vi "FilterSixArray.vi"(11 "DesiredFM_FF":dbl[](array[numeric])) -> (3 "appended array":dbl[](array[numeric]))   [LabVIEW 2017]
uses:
  <vilib>/Analysis/3filter.llb/Filter Passband Type.ctl
  <vilib>/ptbypt/NI_PtbyPt.lvlib
  <vilib>/Analysis/NI_AALBase.lvlib
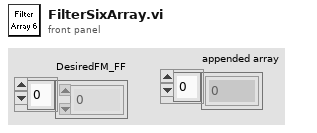
[diagram p1: front panel]
types:
  T1 = typedef "NI_AALBase.lvlib/Filter Passband Type.ctl" = enum32{"Lowpass", "Highpass", "Bandpass", "Bandstop"}
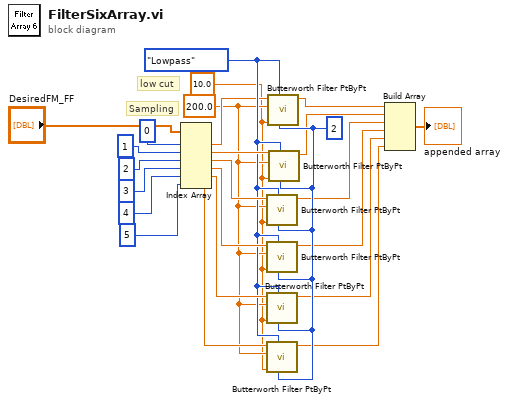
[diagram p0: block diagram]
diagram:
  w8 = 10.0 ("sampling freq: fs")
  w9 = 2 ("order")
  w10 = 200.0 ("sampling freq: fs")
  w12 = Filter_Passband_Type."Lowpass" ("filter type")
  # "Sampling"
  # "low cut"
  n1 = Index Array(array="DesiredFM_FF", index #1=0 ("index"), index #2=1 ("index"), index #3=2 ("index"), index #4=3 ("index"), index #5=4 ("index"), index #6=5 ("index")) -> (element #1=w11:dbl, element #2=w17:dbl, element #3=w16:dbl, element #4=w15:dbl, element #5=w14:dbl, element #6=w13:dbl)
  n2 = call <vilib>:"Butterworth Filter PtByPt.vi"("order"=w9, "filter type"=w12, "low cutoff freq: fl"=w8, "sampling freq: fs"=w10, "x"=w16) -> ("Filtered x"=w5:dbl)  [unwired: 4 in, 1 out]
  n3 = call <vilib>:"Butterworth Filter PtByPt.vi"("order"=w9, "filter type"=w12, "low cutoff freq: fl"=w8, "sampling freq: fs"=w10, "x"=w15) -> ("Filtered x"=w4:dbl)  [unwired: 4 in, 1 out]
  n4 = call <vilib>:"Butterworth Filter PtByPt.vi"("order"=w9, "filter type"=w12, "low cutoff freq: fl"=w8, "sampling freq: fs"=w10, "x"=w14) -> ("Filtered x"=w3:dbl)  [unwired: 4 in, 1 out]
  n5 = call <vilib>:"Butterworth Filter PtByPt.vi"("order"=w9, "filter type"=w12, "low cutoff freq: fl"=w8, "sampling freq: fs"=w10, "x"=w13) -> ("Filtered x"=w2:dbl)  [unwired: 4 in, 1 out]
  n6 = call <vilib>:"Butterworth Filter PtByPt.vi"("order"=w9, "filter type"=w12, "low cutoff freq: fl"=w8, "sampling freq: fs"=w10, "x"=w11) -> ("Filtered x"=w7:dbl)  [unwired: 4 in, 1 out]
  n7 = call <vilib>:"Butterworth Filter PtByPt.vi"("order"=w9, "filter type"=w12, "low cutoff freq: fl"=w8, "sampling freq: fs"=w10, "x"=w17) -> ("Filtered x"=w6:dbl)  [unwired: 4 in, 1 out]
  n8 = Build Array(w7, w6, w5, w4, w3, w2) -> (→"appended array":dbl[])
